vi "FSM.vi"() -> ()   [LabVIEW 2018]
panel:
  out "Initializing":bool
  out "Running":bool
  in  "stop":bool
  in  "Restart":bool
  in  "Start Initializing":bool
  in  "Start Running":bool
  in  "Reset":bool
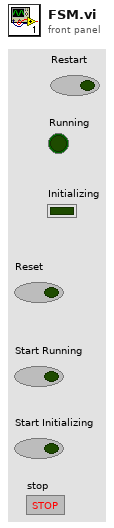
[diagram p1: front panel]
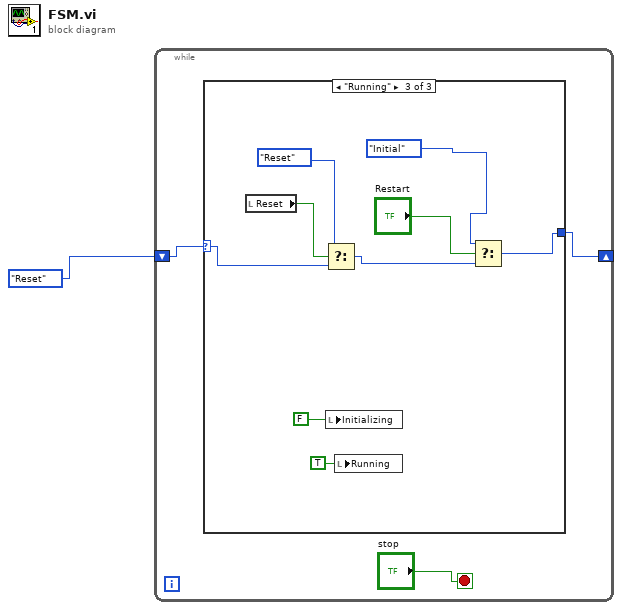
[diagram p0: block diagram]
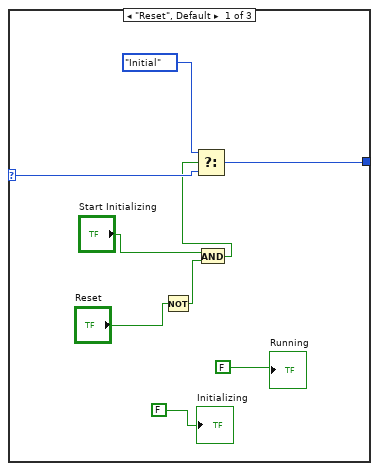
[diagram p2: hidden frame]
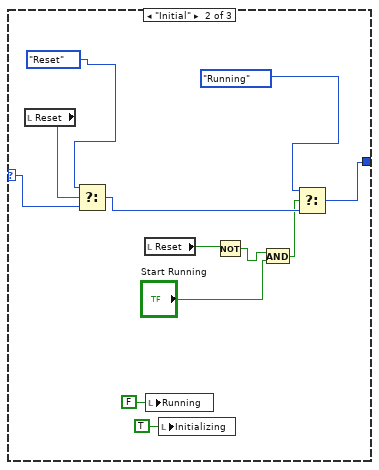
[diagram p3: hidden frame]
diagram:
  n1 = while {
    shift-right: [w2] -> _
    shift-left: enum16{"Reset", "Initial", "Running"}."Reset" -> [w3]
    stop <- "stop" stop-if-true
    n2 = case shown="\"Running\"" w3 {
      selector: w3 -> [w13 w18 w29]
      tunnel: [w8 w25 w30] -> w2
      frame "Reset", Default {
        n3 = Not(x="Reset") -> (.not. x?=w11:bool)
        n4 = And(x="Start Initializing", y=w11) -> (x .and. y?=w12:bool)
        n5 = Select(t=enum16{"Reset", "Initial", "Running"}."Initial", s=w12, f=w13) -> (s? t:f=w8:enum16{"Reset", "Initial", "Running"})
        "Initializing" <- FALSE ("Initializing")
        "Running" <- FALSE ("Running")
      }
      frame "Initial" {
        n6 = local read "Reset"() -> (w19:bool)
        n7 = Select(t=enum16{"Reset", "Initial", "Running"}."Reset", s=w19, f=w18) -> (s? t:f=w24:enum16{"Reset", "Initial", "Running"})
        n8 = local read "Reset"() -> (w23:bool)
        n9 = local write "Running"(FALSE ("Running")) -> ()
        n10 = local write "Initializing"(TRUE ("Initializing")) -> ()
        n11 = Not(x=w23) -> (.not. x?=w22:bool)
        n12 = And(x=w22, y="Start Running") -> (x .and. y?=w20:bool)
        n13 = Select(t=enum16{"Reset", "Initial", "Running"}."Running", s=w20, f=w24) -> (s? t:f=w25:enum16{"Reset", "Initial", "Running"})
      }
      frame "Running" {
        n14 = local read "Reset"() -> (w28:bool)
        n15 = Select(t=enum16{"Reset", "Initial", "Running"}."Reset", s=w28, f=w29) -> (s? t:f=w32:enum16{"Reset", "Initial", "Running"})
        n16 = local write "Initializing"(FALSE) -> ()
        n17 = local write "Running"(TRUE ("Running")) -> ()
        n18 = Select(t=enum16{"Reset", "Initial", "Running"}."Initial", s="Restart", f=w32) -> (s? t:f=w30:enum16{"Reset", "Initial", "Running"})
      }
    }
  }
